vi "error code mapping for polynomial.vi"(11 "error in":i32) -> (3 "error out":i32)   [LabVIEW 2013, in "NI_AALPro.lvlib"]
uses:
  NI_AALPro.lvlib
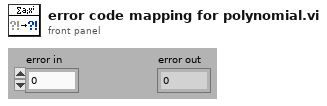
[diagram p1: front panel]
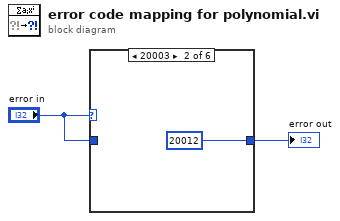
[diagram p0: block diagram]
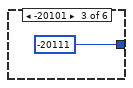
[diagram p3: hidden frame]
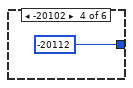
[diagram p4: hidden frame]
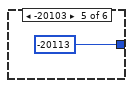
[diagram p5: hidden frame]
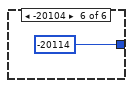
[diagram p6: hidden frame]
diagram:
  n1 = case shown="20003" "error in" {
    tunnel: [w3 20012 ("error in") -20111 ("error in") -20112 ("error in") -20113 ("error in") -20114 ("error in")] -> w2
    tunnel: "error in" -> [w3 _ _ _ _ _]
    frame Default {
    }
    frame 20003 {
    }
    frame -20101 {
    }
    frame -20102 {
    }
    frame -20103 {
    }
    frame -20104 {
    }
  }
  "error out" <- w2
